vi "RT Target.vi"(8 "error in":errorcluster) -> (0 "error out":errorcluster)   [LabVIEW 2017]
doc: "Perform control a DAQ HW in the deterministic mode."
uses:
  <vilib>/Platform/TimedLoop/XDataNode/timing_clust.ctl
  <vilib>/Platform/TimedLoop/XDataNode/nitl_modes.ctl
  <vilib>/Platform/TimedLoop/XDataNode/wakeup.ctl
  RT Loop Status.ctl
  RT Status.ctl
  <vilib>/DAQmx/read.llb/DAQmx Read (Analog 1D DBL NChan 1Samp).vi
  <vilib>/DAQmx/read.llb/DAQmx Read (Digital 1D Bool 1Chan 1Samp).vi
  <vilib>/DAQmx/write.llb/DAQmx Write (Digital 1D Bool 1Chan 1Samp).vi
  <vilib>/DAQmx/write.llb/DAQmx Write (Analog 1D DBL NChan 1Samp).vi
  <vilib>/DAQmx/create/channels.llb/DAQmx Create Channel (AI-Voltage-Basic).vi
  <vilib>/DAQmx/create/channels.llb/DAQmx Create Channel (DI-Digital Input).vi
  <vilib>/DAQmx/create/channels.llb/DAQmx Create Channel (AO-Voltage-Basic).vi
  <vilib>/DAQmx/create/channels.llb/DAQmx Create Channel (AO-Current-Basic).vi
  <vilib>/DAQmx/create/channels.llb/DAQmx Create Channel (DO-Digital Output).vi
  <vilib>/DAQmx/miscellaneous.llb/DAQmx Fill In Error Info.vi
  <vilib>/Platform/TimedLoop/XDataNode/XDataNode.xnode
  <vilib>/Platform/TimedLoop/XDataNode/XDNodeRunTimeDep.lvlib
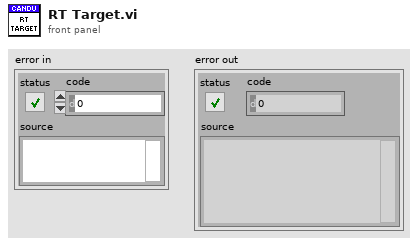
[diagram p1: front panel]
types:
  T1 = typedef "XDNodeRunTimeDep.lvlib/timing_clust.ctl" = cluster{"Expected End [f-1]":u64, "Actual End [f-1]":u64, "Finished Late? [f-1]":bool, "Expected End [i-1]":u64, "Actual End [i-1]":u64, "Finished Late? [i-1]":bool, "Expected Start [i]":u64, "Actual Start [i]":u64, "Expected Start [f]":u64, "Actual Start [f]":u64, "Source Name":string, "Structure Name":string, "Period":i64, "Deadline":i64, "Offset":i64, "Start":i64, "Priority":i32, "Timeout":i32, "Mode":T2, "Wakeup Reason":T3, "Error":errorcluster, "Source Type":string, "Secondary Source Type":string, "Global End Time":u64, "Global Start Time":u64, "Frame Duration":u64, "Iteration Duration":u64, "Assigned CPU":i32, "I/O Scan Engine Mode":u32}
  T2 = typedef "XDNodeRunTimeDep.lvlib/nitl_modes.ctl" = enum32{"No Change", "Process missed periods, maintain original phase", "Discard missed periods, maintain original phase", "Process missed periods, ignore original phase", "Discard missed periods, ignore original phase"}
  T3 = typedef "XDNodeRunTimeDep.lvlib/wakeup.ctl" = enum32{"Normal", "Aborted", "Asynchronous wakeup", "Timing source error", "Timed loop error", "Timeout"}
  T4 = typedef "RT Loop Status.ctl" = cluster{"Duration, us":dbl, "Late Counter":i32, "Timeout, us":u32}
  T5 = typedef "RT Status.ctl" = cluster{"Status TCL1":T4, "Status TCL2":T4, "Status NPL":T4, "Connected?":bool}
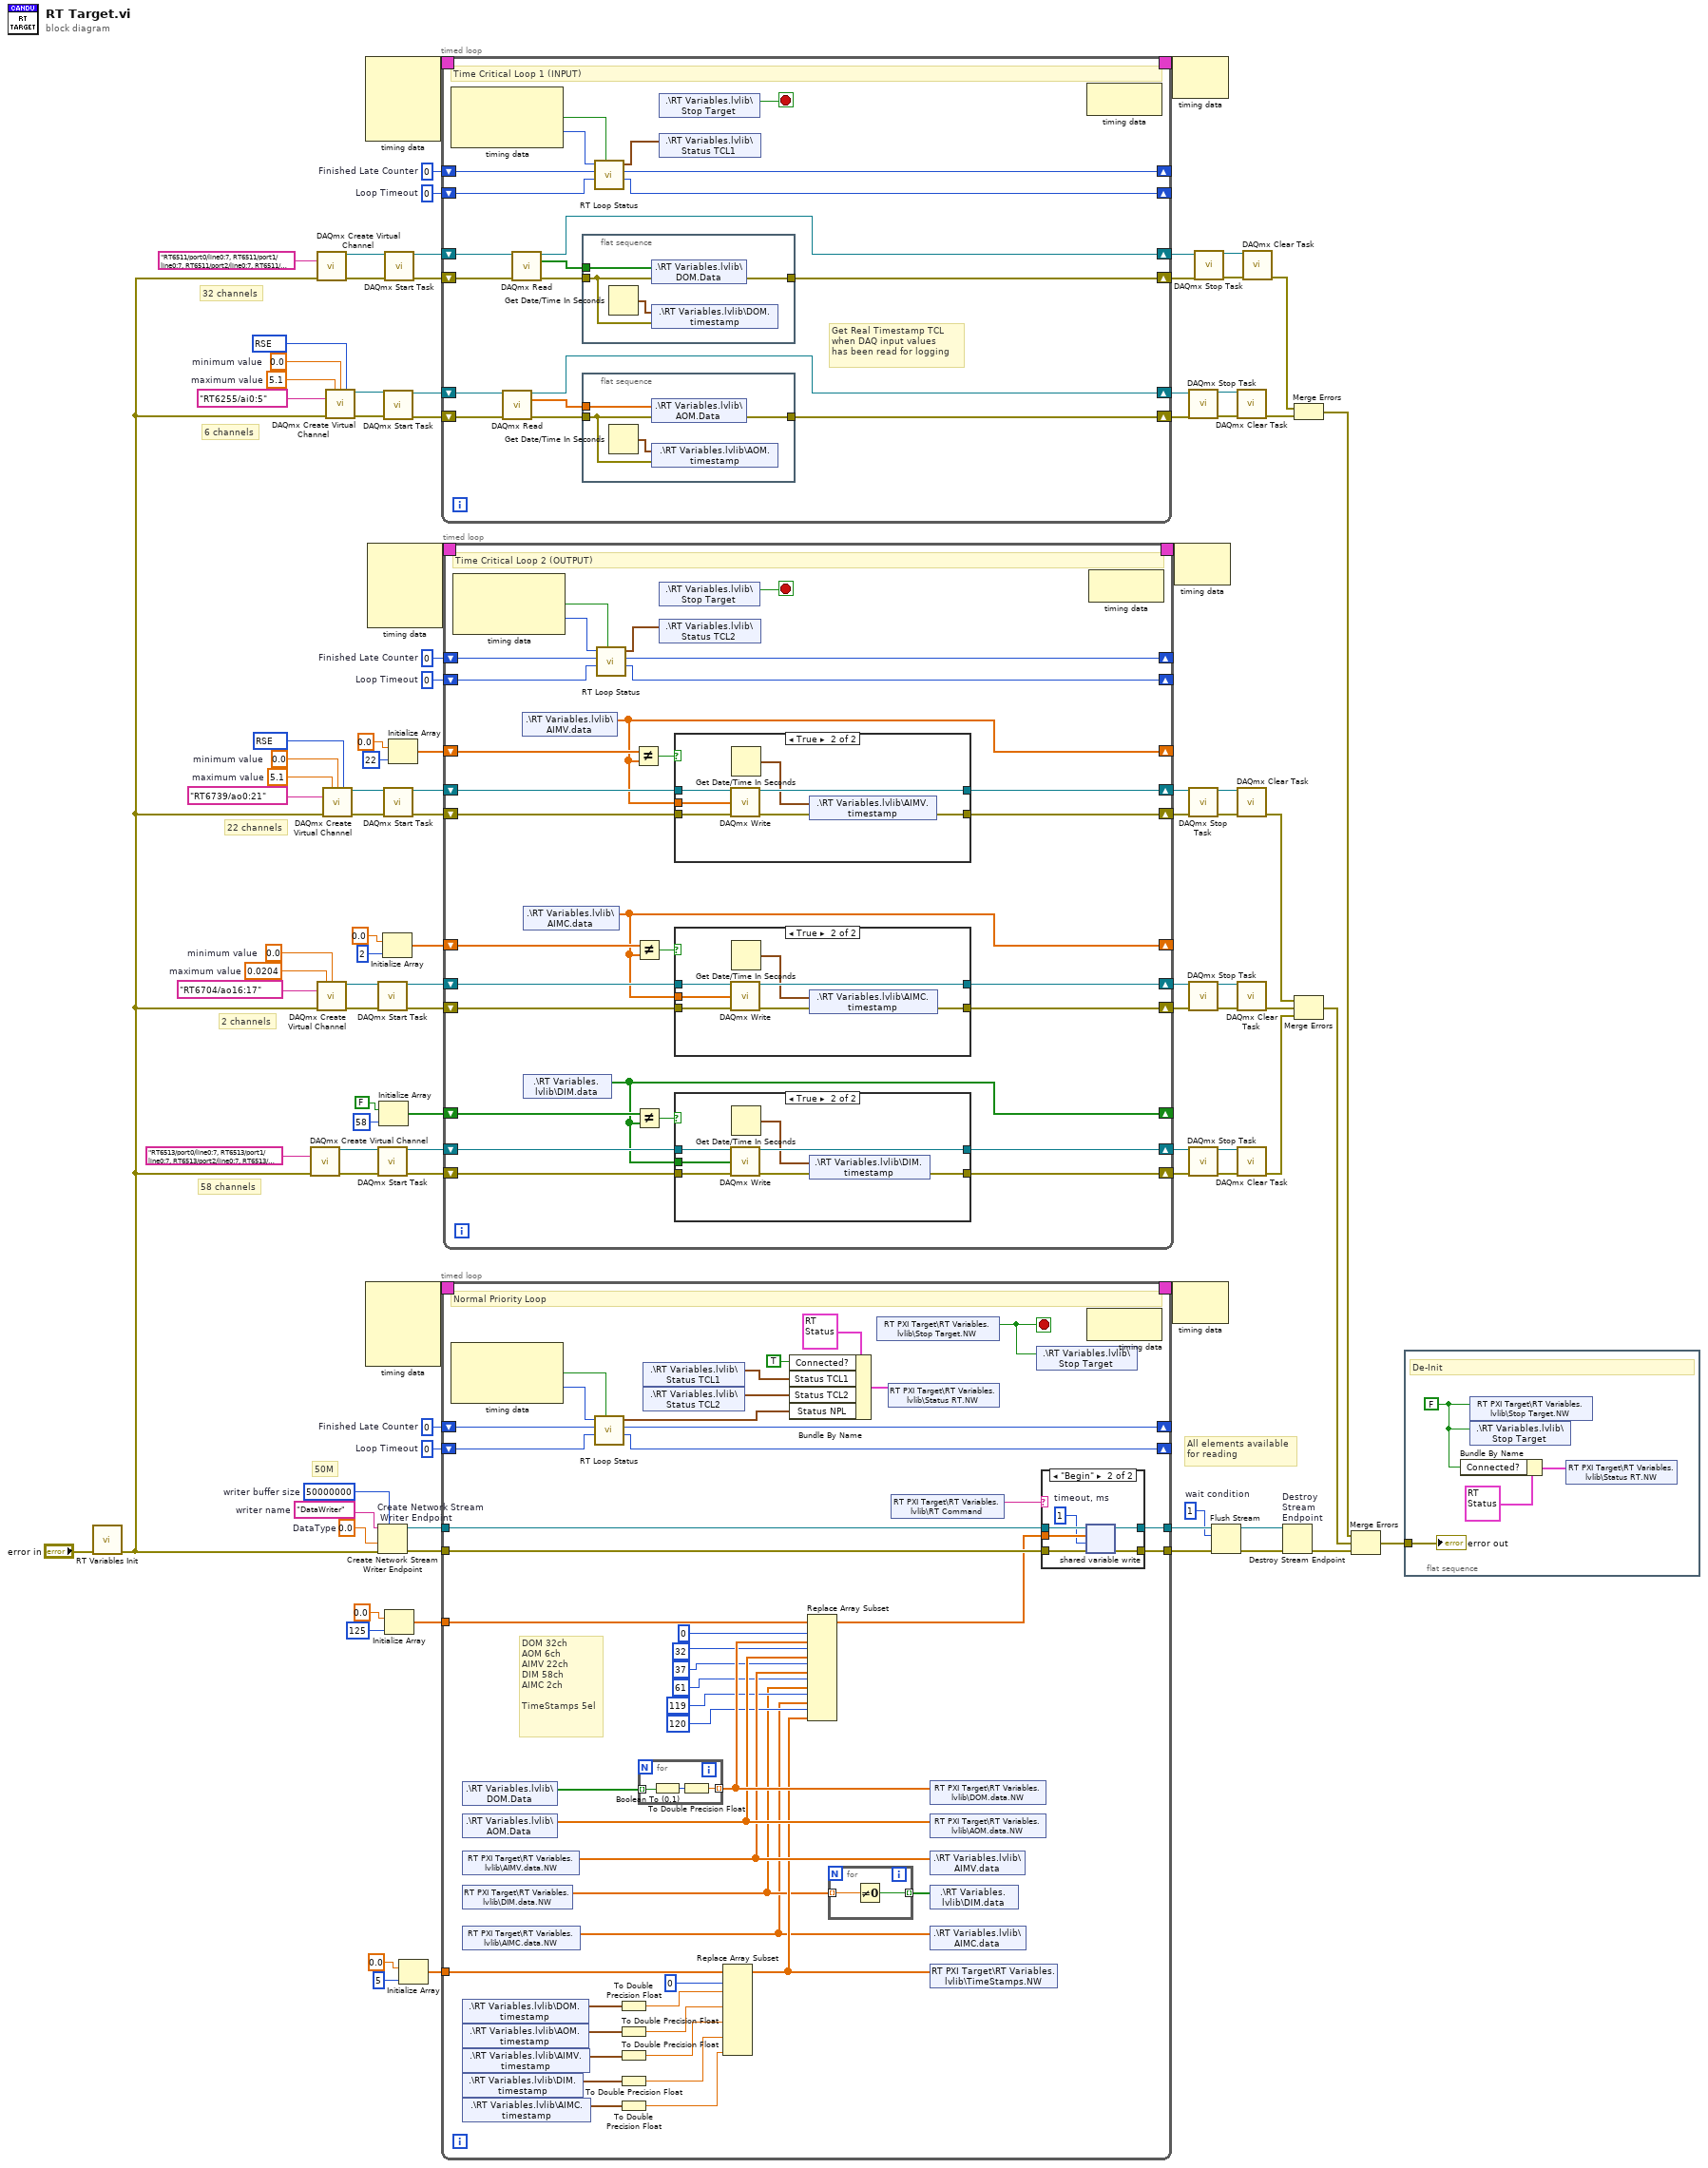
[diagram p0: block diagram]
diagram:
  w13 = u8 1  # wait condition
  w20 = 0.0  # DataType
  w21 = 50000000  # writer buffer size
  w22 = "DataWriter"  # writer name
  w50 = 0.0204  # maximum value
  w51 = 0.0  # minimum value
  w66 = 10083 items=["Default"=-1, "RSE"=10083, "Differential"=10106, "Pseudodifferential"=12529] ("output terminal configuration")
  w64 = 5.1  # maximum value
  w63 = 0.0  # minimum value
  w82 = 10083 items=["Default"=-1, "RSE"=10083, "NRSE"=10078, "Differential"=10106, "Pseudodifferential"=12529] ("input terminal configuration")
  w85 = 5.1  # maximum value
  w86 = 0.0  # minimum value
  w93 = u32 0  # Loop Timeout
  w92 = 0  # Finished Late Counter
  w90 = u32 0  # Loop Timeout
  w91 = 0  # Finished Late Counter
  w94 = u32 0  # Loop Timeout
  w95 = 0  # Finished Late Counter
  # "50M"
  # "All elements available\nfor reading"
  # "58 channels"
  # "2 channels"
  # "22 channels"
  # "32 channels"
  # "6 channels"
  n1 = call "RT Variables Init.vi"("error in (no error)"="error in") -> ("error out"=w2:errorcluster)  [unwired: 9 in, 1 out]
  n2 = call-poly <vilib>:"DAQmx Create Virtual Channel.vi"("lines"=tag "RT6513/port0/line0:7, RT6513/port1/line0:7, RT6513/port2/line0:7, RT6513/port3/line0:7, RT6513/port4/line0:7, RT6513/port5/line0:7, RT6513/port6/line0:7, RT6513/port7/line0:1" ("Ch.Phys"), "error in"=w2) -> ("task out"=w43:refnum<k21>, "error out"=w44:errorcluster)  [unwired: 12 in]
  n3 = call-poly <vilib>:"DAQmx Create Virtual Channel.vi"("lines"=tag "RT6511/port0/line0:7, RT6511/port1/line0:7, RT6511/port2/line0:7, RT6511/port3/line0:7" ("Ch.Phys"), "error in"=w2) -> ("task out"=w89:refnum<k21>, "error out"=w88:errorcluster)  [unwired: 12 in]
  n4 = call-poly <vilib>:"DAQmx Create Virtual Channel.vi"("maximum value"=w50, "minimum value"=w51, "physical channels"=tag "RT6704/ao16:17", "error in"=w2) -> ("task out"=w53:refnum<k21>, "error out"=w52:errorcluster)  [unwired: 10 in]
  n5 = call-poly <vilib>:"DAQmx Create Virtual Channel.vi"("maximum value"=w64, "minimum value"=w63, "output terminal configuration"=w66, "physical channels"=tag "RT6739/ao0:21", "error in"=w2) -> ("task out"=w61:refnum<k21>, "error out"=w62:errorcluster)  [unwired: 9 in]
  n6 = call-poly <vilib>:"DAQmx Create Virtual Channel.vi"("maximum value"=w85, "minimum value"=w86, "input terminal configuration"=w82, "physical channels"=tag "RT6255/ai0:5", "error in"=w2) -> ("task out"=w84:refnum<k21>, "error out"=w83:errorcluster)  [unwired: 9 in]
  n7 = node-c288() -> (w99:T1)  [unwired: 4 in]
  n8 = node-c288() -> (w101:T1)  [unwired: 4 in]
  n9 = node-c288() -> (w97:T1)  [unwired: 4 in]
  n10 = call <vilib>:"DAQmx Start Task.vi"("task/channels in"=w53, "error in"=w52) -> ("task out"=w47:refnum<k21>, "error out"=w46:errorcluster)  [unwired: 12 in]
  n11 = call <vilib>:"DAQmx Start Task.vi"("task/channels in"=w43, "error in"=w44) -> ("task out"=w39:refnum<k21>, "error out"=w38:errorcluster)  [unwired: 12 in]
  n12 = Create Network Stream Writer Endpoint "Create Network Stream\n Writer Endpoint"(7:w21, 8:w2, 9:w20, 11:w22) -> (0:w18:errorcluster, 3:w19:refnum<k21>)  [unwired: 3 in]
  n13 = Initialize Array(FALSE, 58 ("dimension size")) -> (w40:bool[])
  n14 = Initialize Array(0.0, 2 ("dimension size")) -> (w48:dbl[])
  n15 = call <vilib>:"DAQmx Start Task.vi"("task/channels in"=w84, "error in"=w83) -> ("task out"=w78:refnum<k21>, "error out"=w77:errorcluster)  [unwired: 12 in]
  n16 = call <vilib>:"DAQmx Start Task.vi"("task/channels in"=w61, "error in"=w62) -> ("task out"=w57:refnum<k21>, "error out"=w56:errorcluster)  [unwired: 12 in]
  n17 = call <vilib>:"DAQmx Start Task.vi"("task/channels in"=w89, "error in"=w88) -> ("task out"=w80:refnum<k21>, "error out"=w79:errorcluster)  [unwired: 12 in]
  n18 = Initialize Array(0.0, 125 ("dimension size")) -> (w6:dbl[])
  n19 = Initialize Array(0.0, 22 ("dimension size")) -> (w58:dbl[])
  n20 = Initialize Array(0.0, 5 ("dimension size")) -> (w3:dbl[])
  n21 = timed-loop {
    timing: w99 -> [_]
    timing-out: [_] -> w98
    shift-right: [w116] -> _
    shift-left: w92 -> [w119]
    shift-right: [w117] -> _
    shift-left: w93 -> [w118]
    shift-right: [w106] -> w69
    shift-left: w80 -> [w112]
    shift-right: [w107] -> w70
    shift-left: w79 -> [w113]
    shift-right: [w102] -> w71
    shift-left: w78 -> [w111]
    shift-right: [w103] -> w72
    shift-left: w77 -> [w110]
    stop <- w114 stop-if-true
    # "Get Real Timestamp TCL\nwhen DAQ input values\nhas been read for logging"
    # "Time Critical Loop 1 (INPUT)"
    n22 = node-c288() -> (w121:bool, w120:i64)  [unwired: 1 in, 1 out]
    n23 = call-poly <vilib>:"DAQmx Read.vi"("task/channels in"=w111, "error in"=w110) -> ("task out"=w102:refnum<k21>, "data"=w104:dbl[], "error out"=w105:errorcluster)  [unwired: 11 in]
    n24 = call-poly <vilib>:"DAQmx Read.vi"("task/channels in"=w112, "error in"=w113) -> ("task out"=w106:refnum<k21>, "data"=w108:bool[], "error out"=w109:errorcluster)  [unwired: 11 in]
    n25 = flat-sequence {
      tunnel: w109 -> [w128]
      tunnel: w108 -> [w129]
      tunnel: [w126] -> w107
      frame #0 {
        n26 = Get Date/Time In Seconds() -> (seconds since 1Jan1904=w127:timestamp)
        n27 = shared-variable ".\\RT Variables.lvlib\\DOM.Data"(w129, error in=w128) -> (error out=w126:errorcluster)
        n28 = shared-variable ".\\RT Variables.lvlib\\DOM.timestamp"(w127, error in=w128) -> ()  [unwired: 1 out]
      }
    }
    n29 = flat-sequence {
      tunnel: w105 -> [w124]
      tunnel: w104 -> [w125]
      tunnel: [w122] -> w103
      frame #0 {
        n30 = Get Date/Time In Seconds() -> (seconds since 1Jan1904=w123:timestamp)
        n31 = shared-variable ".\\RT Variables.lvlib\\AOM.Data"(w125, error in=w124) -> (error out=w122:errorcluster)
        n32 = shared-variable ".\\RT Variables.lvlib\\AOM.timestamp"(w123, error in=w124) -> ()  [unwired: 1 out]
      }
    }
    n33 = call "RT Loop Status.vi"("Finished Late?"=w121, "Loop Timeout in"=w118, "Finished Late Counter in"=w119, "Iteration Duration"=w120) -> ("Loop Timeout out"=w117:u32, "Finished Late Counter out"=w116:i32, "Loop Status"=w115:T4)  [unwired: 4 in, 1 out]
    n34 = shared-variable ".\\RT Variables.lvlib\\Stop Target"() -> (w114:bool)  [unwired: 1 in, 1 out]
    n35 = shared-variable ".\\RT Variables.lvlib\\Status TCL1"(w115) -> ()  [unwired: 1 in, 1 out]
    n36 = node-c288() -> ()  [unwired: 1 in, 1 out]
  }
  n37 = timed-loop {
    timing: w101 -> [_]
    timing-out: [_] -> w100
    shift-right: [w169] -> _
    shift-left: w95 -> [w172]
    shift-right: [w170] -> _
    shift-left: w94 -> [w171]
    tunnel: w19 -> [w166]
    tunnel: w18 -> [w165]
    tunnel: [w163] -> w15
    tunnel: [w162] -> w14
    tunnel: w6 -> [w149]
    tunnel: w3 -> [w154]
    stop <- w179 stop-if-true
    # "DOM 32ch\nAOM 6ch\nAIMV 22ch\nDIM 58ch\nAIMC 2ch\n\nTimeStamps 5el"
    # "Normal Priority Loop"
    n38 = node-c288() -> (w174:bool, w173:i64)  [unwired: 1 in, 1 out]
    n39 = shared-variable ".\\RT Variables.lvlib\\DOM.Data"() -> (w156:bool[])  [unwired: 1 in, 1 out]
    n40 = shared-variable ".\\RT Variables.lvlib\\AOM.Data"() -> (w146:dbl[])  [unwired: 1 in, 1 out]
    n41 = shared-variable "RT PXI Target\\RT Variables.lvlib\\AIMV.data.NW"() -> (w145:dbl[])  [unwired: 1 in, 1 out]
    n42 = shared-variable "RT PXI Target\\RT Variables.lvlib\\DIM.data.NW"() -> (w135:dbl[])  [unwired: 1 in, 1 out]
    n43 = shared-variable "RT PXI Target\\RT Variables.lvlib\\AIMC.data.NW"() -> (w134:dbl[])  [unwired: 1 in, 1 out]
    n44 = shared-variable ".\\RT Variables.lvlib\\DOM.timestamp"() -> (w161:timestamp)  [unwired: 1 in, 1 out]
    n45 = shared-variable ".\\RT Variables.lvlib\\AOM.timestamp"() -> (w160:timestamp)  [unwired: 1 in, 1 out]
    n46 = shared-variable ".\\RT Variables.lvlib\\AIMV.timestamp"() -> (w159:timestamp)  [unwired: 1 in, 1 out]
    n47 = shared-variable ".\\RT Variables.lvlib\\DIM.timestamp"() -> (w157:timestamp)  [unwired: 1 in, 1 out]
    n48 = shared-variable ".\\RT Variables.lvlib\\AIMC.timestamp"() -> (w158:timestamp)  [unwired: 1 in, 1 out]
    n49 = call "RT Loop Status.vi"("Finished Late?"=w174, "Loop Timeout in"=w171, "Finished Late Counter in"=w172, "Iteration Duration"=w173) -> ("Loop Timeout out"=w170:u32, "Finished Late Counter out"=w169:i32, "Loop Status"=w168:T4)  [unwired: 4 in, 1 out]
    n50 = To Double Precision Float(number=w161) -> (double precision float=w152:dbl)
    n51 = To Double Precision Float(number=w160) -> (double precision float=w151:dbl)
    n52 = To Double Precision Float(number=w159) -> (double precision float=w150:dbl)
    n53 = To Double Precision Float(number=w157) -> (double precision float=w137:dbl)
    n54 = To Double Precision Float(number=w158) -> (double precision float=w136:dbl)
    n55 = for {
      tunnel: w156 -> [w184] mode=indexing
      tunnel: [w182] -> w147 mode=indexing
      n56 = Boolean To (0,1)(Boolean=w184) -> (0, 1=w183:i16)
      n57 = To Double Precision Float(number=w183) -> (double precision float=w182:dbl)
    }
    n58 = shared-variable ".\\RT Variables.lvlib\\Status TCL1"() -> (w178:T4)  [unwired: 1 in, 1 out]
    n59 = shared-variable ".\\RT Variables.lvlib\\Status TCL2"() -> (w177:T4)  [unwired: 1 in, 1 out]
    n60 = Replace Array Subset(array=w154, new element #1=w152, index #1=0 ("index"), new element #2=w151, new element #3=w150, new element #4=w137, new element #5=w136) -> (w144:dbl[])  [unwired: 4 in]
    n61 = Bundle By Name(cluster=T5 {"Status TCL1"={"Duration, us"=0.0, "Late Counter"=0, "Timeout, us"=0}, "Status TCL2"={"Duration, us"=0.0, "Late Counter"=0, "Timeout, us"=0}, "Status NPL"={"Duration, us"=0.0, "Late Counter"=0, "Timeout, us"=0}, "Connected?"=FALSE} ("RT Status"), "Connected?"=TRUE, "Status TCL1"=w178, "Status TCL2"=w177, "Status NPL"=w168) -> (w175:T5)
    n62 = Replace Array Subset(array=w149, new element #1=w147, index #1=0 ("index"), new element #2=w146, index #2=32 ("index"), new element #3=w145, index #3=37 ("index"), new element #4=w135, index #4=61 ("index"), new element #5=w134, index #5=119 ("index"), new element #6=w144, index #6=120 ("index")) -> (w143:dbl[])
    n63 = for {
      tunnel: w135 -> [w181] mode=indexing
      tunnel: [w180] -> w155 mode=indexing
      n64 = Not Equal To 0?(x=w181) -> (x != 0?=w180:bool)
    }
    n65 = shared-variable "RT PXI Target\\RT Variables.lvlib\\Stop Target.NW"() -> (w179:bool)  [unwired: 1 in, 1 out]
    n66 = shared-variable "RT PXI Target\\RT Variables.lvlib\\Status RT.NW"(w175) -> ()  [unwired: 1 in, 1 out]
    n67 = shared-variable "RT PXI Target\\RT Variables.lvlib\\RT Command"() -> (w164:string)  [unwired: 1 in, 1 out]
    n68 = shared-variable "RT PXI Target\\RT Variables.lvlib\\DOM.data.NW"(w147) -> ()  [unwired: 1 in, 1 out]
    n69 = shared-variable "RT PXI Target\\RT Variables.lvlib\\AOM.data.NW"(w146) -> ()  [unwired: 1 in, 1 out]
    n70 = shared-variable ".\\RT Variables.lvlib\\AIMV.data"(w145) -> ()  [unwired: 1 in, 1 out]
    n71 = shared-variable ".\\RT Variables.lvlib\\DIM.data"(w155) -> ()  [unwired: 1 in, 1 out]
    n72 = shared-variable ".\\RT Variables.lvlib\\AIMC.data"(w134) -> ()  [unwired: 1 in, 1 out]
    n73 = shared-variable "RT PXI Target\\RT Variables.lvlib\\TimeStamps.NW"(w144) -> ()  [unwired: 1 in, 1 out]
    n74 = shared-variable ".\\RT Variables.lvlib\\Stop Target"(w179) -> ()  [unwired: 1 in, 1 out]
    n75 = case shown="\"Begin\"" w164 {
      tunnel: w166 -> [w186 w192]
      tunnel: w165 -> [w185 w191]
      tunnel: w143 -> [_ w190]
      tunnel: [w186 w189] -> w162
      tunnel: [w185 w188] -> w163
      frame "Idle", Default {
      }
      frame "Begin" {
        w187 = 1  # timeout, ms
        n76 = shared-variable-write(w192, w191, w190, w187) -> (w189:refnum<k21>, w188:errorcluster)  [unwired: 1 out]
      }
    }
    n77 = node-c288() -> ()  [unwired: 1 in, 1 out]
  }
  n78 = timed-loop {
    timing: w97 -> [_]
    timing-out: [_] -> w96
    shift-right: [w220] -> _
    shift-left: w91 -> [w223]
    shift-right: [w221] -> _
    shift-left: w90 -> [w222]
    shift-right: [w211] -> _
    shift-left: w58 -> [w217]
    shift-right: [w213] -> w26
    shift-left: w57 -> [w216]
    shift-right: [w212] -> w27
    shift-left: w56 -> [w215]
    shift-right: [w204] -> _
    shift-left: w48 -> [w209]
    shift-right: [w206] -> w28
    shift-left: w47 -> [w208]
    shift-right: [w205] -> w29
    shift-left: w46 -> [w207]
    shift-right: [w199] -> _
    shift-left: w40 -> [w202]
    shift-right: [w198] -> w31
    shift-left: w39 -> [w200]
    shift-right: [w197] -> w30
    shift-left: w38 -> [w201]
    stop <- w218 stop-if-true
    # "Time Critical Loop 2 (OUTPUT)"
    n79 = node-c288() -> (w225:bool, w224:i64)  [unwired: 1 in, 1 out]
    n80 = shared-variable ".\\RT Variables.lvlib\\AIMV.data"() -> (w211:dbl[])  [unwired: 1 in, 1 out]
    n81 = shared-variable ".\\RT Variables.lvlib\\AIMC.data"() -> (w204:dbl[])  [unwired: 1 in, 1 out]
    n82 = shared-variable ".\\RT Variables.lvlib\\DIM.data"() -> (w199:bool[])  [unwired: 1 in, 1 out]
    n83 = call "RT Loop Status.vi"("Finished Late?"=w225, "Loop Timeout in"=w222, "Finished Late Counter in"=w223, "Iteration Duration"=w224) -> ("Loop Timeout out"=w221:u32, "Finished Late Counter out"=w220:i32, "Loop Status"=w219:T4)  [unwired: 4 in, 1 out]
    n84 = Not Equal?(x=w217, y=w211) -> (x != y?=w214:bool)
    n85 = Not Equal?(x=w209, y=w204) -> (x != y?=w210:bool)
    n86 = Not Equal?(x=w202, y=w199) -> (x != y?=w203:bool)
    n87 = shared-variable ".\\RT Variables.lvlib\\Stop Target"() -> (w218:bool)  [unwired: 1 in, 1 out]
    n88 = shared-variable ".\\RT Variables.lvlib\\Status TCL2"(w219) -> ()  [unwired: 1 in, 1 out]
    n89 = case shown="True" w214 {
      tunnel: w216 -> [w245 w252]
      tunnel: w215 -> [w244 w251]
      tunnel: w211 -> [_ w250]
      tunnel: [w244 w248] -> w212
      tunnel: [w245 w247] -> w213
      frame False {
      }
      frame True {
        n90 = call-poly <vilib>:"DAQmx Write.vi"("task/channels in"=w252, "data"=w250, "error in"=w251) -> ("task out"=w247:refnum<k21>, "error out"=w249:errorcluster)  [unwired: 10 in, 1 out]
        n91 = Get Date/Time In Seconds() -> (seconds since 1Jan1904=w246:timestamp)
        n92 = shared-variable ".\\RT Variables.lvlib\\AIMV.timestamp"(w246, error in=w249) -> (error out=w248:errorcluster)
      }
    }
    n93 = case shown="True" w210 {
      tunnel: w208 -> [w236 w243]
      tunnel: w207 -> [w235 w242]
      tunnel: w204 -> [_ w241]
      tunnel: [w235 w239] -> w205
      tunnel: [w236 w238] -> w206
      frame False {
      }
      frame True {
        n94 = call-poly <vilib>:"DAQmx Write.vi"("task/channels in"=w243, "data"=w241, "error in"=w242) -> ("task out"=w238:refnum<k21>, "error out"=w240:errorcluster)  [unwired: 10 in, 1 out]
        n95 = Get Date/Time In Seconds() -> (seconds since 1Jan1904=w237:timestamp)
        n96 = shared-variable ".\\RT Variables.lvlib\\AIMC.timestamp"(w237, error in=w240) -> (error out=w239:errorcluster)
      }
    }
    n97 = case shown="True" w203 {
      tunnel: w200 -> [w227 w234]
      tunnel: w201 -> [w226 w233]
      tunnel: w199 -> [_ w228]
      tunnel: [w226 w231] -> w197
      tunnel: [w227 w230] -> w198
      frame False {
      }
      frame True {
        n98 = call-poly <vilib>:"DAQmx Write.vi"("task/channels in"=w234, "data"=w228, "error in"=w233) -> ("task out"=w230:refnum<k21>, "error out"=w232:errorcluster)  [unwired: 10 in, 1 out]
        n99 = Get Date/Time In Seconds() -> (seconds since 1Jan1904=w229:timestamp)
        n100 = shared-variable ".\\RT Variables.lvlib\\DIM.timestamp"(w229, error in=w232) -> (error out=w231:errorcluster)
      }
    }
    n101 = node-c288() -> ()  [unwired: 1 in, 1 out]
  }
  n102 = node-c288(w98) -> ()  [unwired: 1 out]
  n103 = node-c288(w100) -> ()  [unwired: 1 out]
  n104 = node-c288(w96) -> ()  [unwired: 1 out]
  n105 = call <vilib>:"DAQmx Stop Task.vi"("task/channels in"=w71, "error in"=w72) -> ("task out"=w74:refnum<k21>, "error out"=w73:errorcluster)  [unwired: 12 in]
  n106 = call <vilib>:"DAQmx Stop Task.vi"("task/channels in"=w26, "error in"=w27) -> ("task out"=w36:refnum<k21>, "error out"=w37:errorcluster)  [unwired: 12 in]
  n107 = call <vilib>:"DAQmx Stop Task.vi"("task/channels in"=w28, "error in"=w29) -> ("task out"=w35:refnum<k21>, "error out"=w34:errorcluster)  [unwired: 12 in]
  n108 = call <vilib>:"DAQmx Stop Task.vi"("task/channels in"=w31, "error in"=w30) -> ("task out"=w32:refnum<k21>, "error out"=w33:errorcluster)  [unwired: 12 in]
  n109 = call <vilib>:"DAQmx Stop Task.vi"("task/channels in"=w69, "error in"=w70) -> ("task out"=w75:refnum<k21>, "error out"=w76:errorcluster)  [unwired: 12 in]
  n110 = Flush Stream(8:w15, 10:w13, 11:w14) -> (0:w16:errorcluster, 3:w17:refnum<k21>)  [unwired: 1 in, 1 out]
  n111 = call <vilib>:"DAQmx Clear Task.vi"("task in"=w74, "error in"=w73) -> ("error out"=w68:errorcluster)  [unwired: 13 in]
  n112 = call <vilib>:"DAQmx Clear Task.vi"("task in"=w36, "error in"=w37) -> ("error out"=w24:errorcluster)  [unwired: 13 in]
  n113 = call <vilib>:"DAQmx Clear Task.vi"("task in"=w35, "error in"=w34) -> ("error out"=w25:errorcluster)  [unwired: 13 in]
  n114 = call <vilib>:"DAQmx Clear Task.vi"("task in"=w32, "error in"=w33) -> ("error out"=w23:errorcluster)  [unwired: 13 in]
  n115 = call <vilib>:"DAQmx Clear Task.vi"("task in"=w75, "error in"=w76) -> ("error out"=w67:errorcluster)  [unwired: 13 in]
  n116 = Destroy Stream Endpoint "Destroy \nStream \nEndpoint"(8:w16, 11:w17) -> (0:w12:errorcluster)
  n117 = Merge Errors(w67, w68) -> (w10:errorcluster)
  n118 = Merge Errors(w24, w25, w23) -> (w11:errorcluster)
  n119 = Merge Errors(w10, w11, w12) -> (w9:errorcluster)
  n120 = flat-sequence {
    tunnel: w9 -> [w257]
    frame #0 {
      w258 = FALSE
      # "De-Init"
      n121 = Bundle By Name(cluster=T5 {"Status TCL1"={"Duration, us"=0.0, "Late Counter"=0, "Timeout, us"=0}, "Status TCL2"={"Duration, us"=0.0, "Late Counter"=0, "Timeout, us"=0}, "Status NPL"={"Duration, us"=0.0, "Late Counter"=0, "Timeout, us"=0}, "Connected?"=FALSE} ("RT Status"), "Connected?"=w258) -> (w259:T5)
      n122 = shared-variable "RT PXI Target\\RT Variables.lvlib\\Stop Target.NW"(w258) -> ()  [unwired: 1 in, 1 out]
      n123 = shared-variable ".\\RT Variables.lvlib\\Stop Target"(w258) -> ()  [unwired: 1 in, 1 out]
      n124 = shared-variable "RT PXI Target\\RT Variables.lvlib\\Status RT.NW"(w259) -> ()  [unwired: 1 in, 1 out]
      "error out" <- w257
    }
  }
